vi "PRIME Telescope Send Stop.vi"(8 "error in (no error)":errorcluster, 11 "connection ID":refnum<k5>) -> (0 "error out":errorcluster)   [LabVIEW 2021, in "PRIME Telescope.lvclass"]
uses:
  PRIME Telescope.lvclass
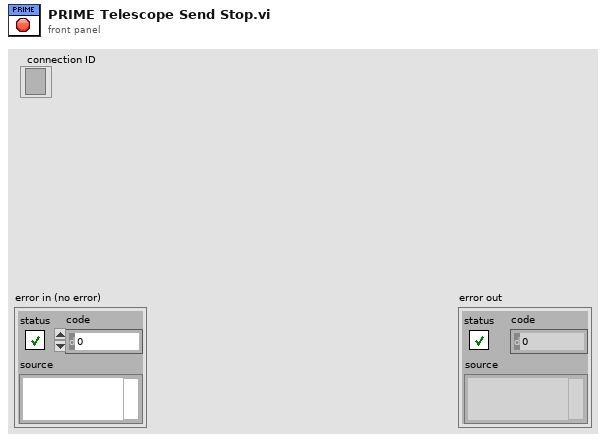
[diagram p1: front panel]
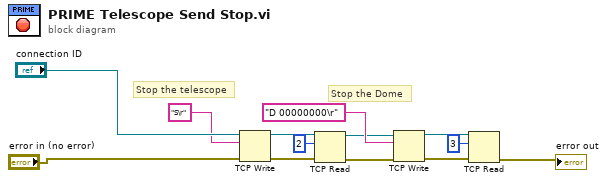
[diagram p0: block diagram]
diagram:
  # "Stop the Dome"
  # "Stop the telescope"
  n1 = TCP Write(connection ID="connection ID", data in="S\r", error in (no error)="error in (no error)") -> (connection ID out=w12:refnum<k5>, error out=w13:errorcluster)  [unwired: 1 in, 1 out]
  n2 = TCP Read(connection ID=w12, bytes to read=2, error in (no error)=w13) -> (connection ID out=w2:refnum<k5>, error out=w3:errorcluster)  [unwired: 2 in, 1 out]
  n3 = TCP Write(connection ID=w2, data in="D 00000000\r", error in (no error)=w3) -> (connection ID out=w5:refnum<k5>, error out=w4:errorcluster)  [unwired: 1 in, 1 out]
  n4 = TCP Read(connection ID=w5, bytes to read=3, error in (no error)=w4) -> (error out=→"error out":errorcluster)  [unwired: 2 in, 2 out]
